vi "Read_lastSequenceId.vi"(8 "error in (no error)":errorcluster, 11 "TcpServerCmd in":refnum<class "TcpServerCmd.lvclass">) -> (0 "error out":errorcluster, 2 "lastSequenceId":i32, 3 "TcpServerCmd out":refnum<class "TcpServerCmd.lvclass">)   [LabVIEW 2018, in "TcpServerCmd.lvclass"]
doc: "Read the last sequenceId sent by TCP Client."
uses:
  TcpServerCmd.lvclass
  TcpServerCmd.lvclass/TcpServerCmd.ctl
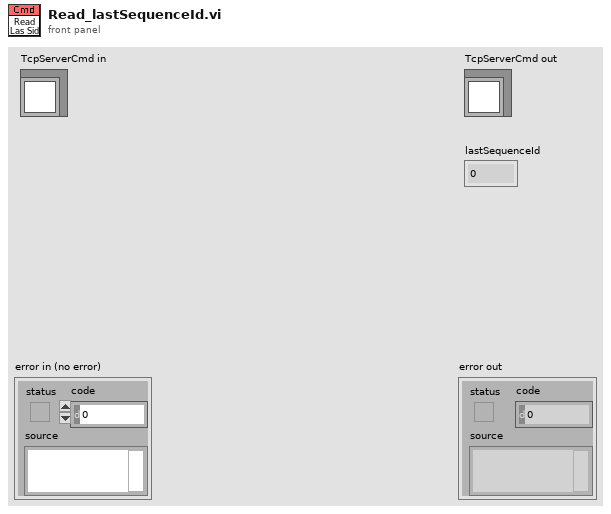
[diagram p1: front panel]
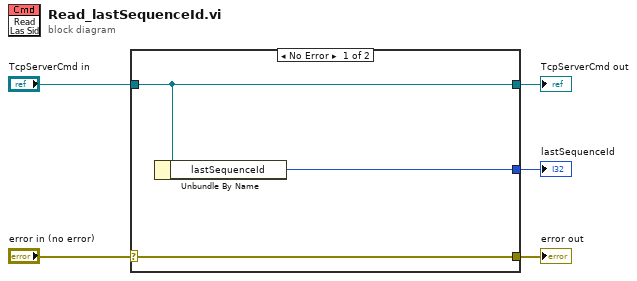
[diagram p0: block diagram]
diagram:
  n1 = case shown="No Error" "error in (no error)" {
    selector: "error in (no error)" -> [w8 w9]
    tunnel: [w8 w9] -> w4
    tunnel: [w7 w10] -> w2
    tunnel: "TcpServerCmd in" -> [w7 w10]
    tunnel: [w6 _] -> w1
    frame No Error {
      n2 = Unbundle By Name(w7) -> ("lastSequenceId"=w6:i32)
    }
    frame Error {
    }
  }
  "error out" <- w4
  "TcpServerCmd out" <- w2
  "lastSequenceId" <- w1
